vi "AuMT8852B EDER Signal Generator Configuration.vi"(5 "Settings":T1={"Modulation Scheme"=enum."PI4", "Pattern"=enum."PRBS9", "TX/RX frequency"=0.0, "Frequency units"=enum."MHz", "Power (dBm)"=0.0, "RF state"=enum."RF on"} {"Power (dBm)" format="%.2f"}, 7 "Set/Get (Set)":enum16{"Set", "Get"}(ring), 8 "error in (no error)":errorcluster, 11 "VISA session":refnum<visa-resource-name>) -> (0 "error out":errorcluster, 2 "error code":i32, 3 "VISA session out":refnum<visa-resource-name>, 4 "Settings out":T1={"Modulation Scheme"=enum."PI4", "Pattern"=enum."PRBS9", "TX/RX frequency"=0.0, "Frequency units"=enum."MHz", "Power (dBm)"=0.0, "RF state"=enum."RF on"} {"Power (dBm)" format="%.2f"})   [LabVIEW 2017]
doc: "Anritsu MT8852B Bluetooth Tester\n\nConfigures the EDR Signal Generator mode. To enter Signal Generator mode, use the Operation Mode command.\n\nINPUTS\nSet/Get - whether to send or retrieve the parameters.\nSettings - new parameters of the signal generator mode.\n\nINPUTS\nSettings out - current parameters of the signal generator mode."
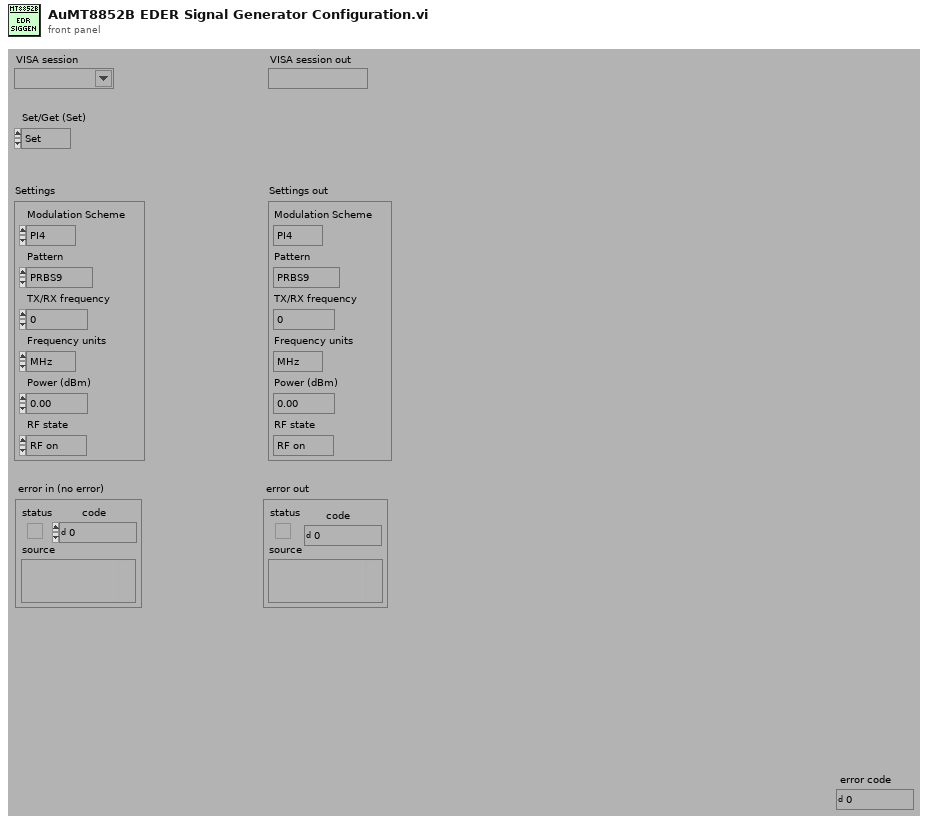
[diagram p1: front panel]
types:
  T1 = cluster{"Modulation Scheme":enum16{"PI4", "8DPSK"}, "Pattern":enum16{"PRBS9", "PRBS15"}, "TX/RX frequency":dbl, "Frequency units":enum16{"Channel", "MHz"}, "Power (dBm)":dbl, "RF state":enum16{"RF off", "RF on"}}
  T2 = enum16{"Simulate", "Range check", "Cache", "Query instrument status"}
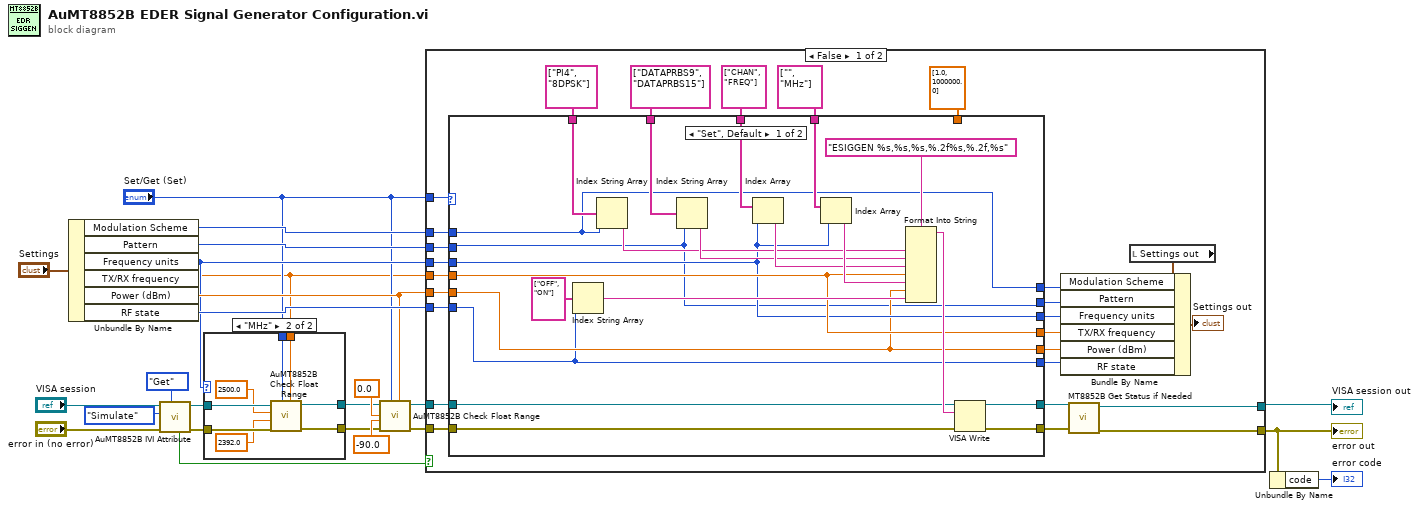
[diagram p0: block diagram]
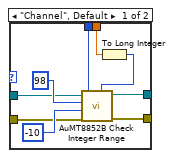
[diagram p2: hidden frame]
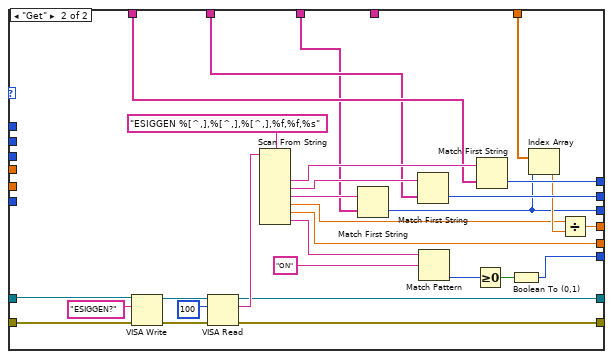
[diagram p3: hidden frame]
diagram:
  n1 = Unbundle By Name("Settings") -> ("Modulation Scheme"=w14:enum16{"PI4", "8DPSK"}, "Pattern"=w13:enum16{"PRBS9", "PRBS15"}, "Frequency units"=w3:enum16{"Channel", "MHz"}, "TX/RX frequency"=w1:dbl, "Power (dBm)"=w11:dbl, "RF state"=w12:enum16{"RF off", "RF on"})
  n2 = call <instrlib>:"AuMT8852B IVI Attribute.vi"("Set/Get (Set)"=enum16{"Set", "Get"}."Get", "error in (no error)"="error in (no error)", "Flag (Simulate)"=T2."Simulate", "VISA session"="VISA session") -> ("error out"=w7:errorcluster, "VISA session out"=w4:refnum<visa-resource-name>, "Value out"=w18:bool)  [unwired: 5 in]
  n3 = case shown="\"MHz\"" w3 {
    tunnel: w7 -> [w31 w41]
    tunnel: [w30 w40] -> w6
    tunnel: [w29 w39] -> w5
    tunnel: w4 -> [w28 w38]
    tunnel: "Set/Get (Set)" -> [w27 w35]
    tunnel: w1 -> [w26 w34]
    frame "Channel", Default {
      n4 = To Long Integer(number=w26) -> (32bit integer=w25:i32)
      n5 = call <instrlib>:"AuMT8852B Check Integer Range.vi"("Value (0)"=w25, "Set/Get (Set)"=w27, "error in (no error)"=w31, "Lower limit (-1)"=-10, "Upper limit (1)"=98, "VISA session"=w28) -> ("error out"=w30:errorcluster, "VISA session out"=w29:refnum<visa-resource-name>)  [unwired: 4 in]
    }
    frame "MHz" {
      n6 = call <instrlib>:"AuMT8852B Check Float Range.vi"("Value (0)"=w34, "Set/Get (Set)"=w35, "error in (no error)"=w41, "Lower limit (-1)"=2392.0, "Upper limit (1)"=2500.0, "VISA session"=w38) -> ("error out"=w40:errorcluster, "VISA session out"=w39:refnum<visa-resource-name>)  [unwired: 4 in]
    }
  }
  n7 = call <instrlib>:"AuMT8852B Check Float Range.vi"("Value (0)"=w11, "Set/Get (Set)"="Set/Get (Set)", "error in (no error)"=w6, "Lower limit (-1)"=-90.0, "Upper limit (1)"=0.0, "VISA session"=w5) -> ("error out"=w17:errorcluster, "VISA session out"=w16:refnum<visa-resource-name>)  [unwired: 4 in]
  n8 = case shown="False" w18 {
    tunnel: [w66 w120] -> w8
    tunnel: [w67 w119] -> w9
    tunnel: w17 -> [w51 w119]
    tunnel: w16 -> [w50 w120]
    tunnel: w3 -> [w49 _]
    tunnel: "Set/Get (Set)" -> [w48 _]
    tunnel: w14 -> [w47 _]
    tunnel: w13 -> [w46 _]
    tunnel: w1 -> [w45 _]
    tunnel: w11 -> [w44 _]
    tunnel: w12 -> [w43 _]
    frame False {
      n9 = case shown="\"Set\", Default" w48 {
        tunnel: [w89 w106] -> w52
        tunnel: [w88 w105] -> w53
        tunnel: [w72 w113] -> w61
        tunnel: [w71 w93] -> w60
        tunnel: [w70 w108] -> w64
        tunnel: [w69 w104] -> w65
        tunnel: string[] ["PI4", "8DPSK"] -> [w76 w96]
        tunnel: string[] ["DATAPRBS9", "DATAPRBS15"] -> [w75 w95]
        tunnel: string[] ["CHAN", "FREQ"] ("Array Constant") -> [w80 w94]
        tunnel: string[] ["", "MHz"] ("Array Constant") -> [w82 _]
        tunnel: [w74 w101] -> w62
        tunnel: dbl[] [1.0, 1000000.0] ("Array Constant") -> [_ w100]
        tunnel: [w73 w90] -> w63
        tunnel: w51 -> [w85 w92]
        tunnel: w50 -> [w84 w91]
        tunnel: w49 -> [w73 _]
        tunnel: w47 -> [w69 _]
        tunnel: w46 -> [w70 _]
        tunnel: w45 -> [w74 _]
        tunnel: w44 -> [w72 _]
        tunnel: w43 -> [w71 _]
        frame "Set", Default {
          n10 = Index String Array(1:w71, 2:string[] ["OFF", "ON"]) -> (0:w83:string)  [unwired: 1 in]
          n11 = Index String Array(1:w69, 2:w76) -> (0:w77:string)  [unwired: 1 in]
          n12 = Index String Array(1:w70, 2:w75) -> (0:w78:string)  [unwired: 1 in]
          n13 = Index Array(array=w80, index=w73) -> (element=w79:string)
          n14 = Index Array(array=w82, index=w73) -> (element=w81:string)
          n15 = Format Into String(format string="ESIGGEN %s,%s,%s,%.2f%s,%.2f,%s" ("Format String"), w77, w78, w79, w74, w81, w72, w83) -> (resulting string=w86:string)  [unwired: 2 in, 1 out]
          n16 = VISA Write(VISA resource name=w84, write buffer=w86, error in (no error)=w85) -> (VISA resource name out=w89:refnum<visa-resource-name>, error out=w88:errorcluster)  [unwired: 1 out]
        }
        frame "Get" {
          n17 = VISA Write(VISA resource name=w91, write buffer="ESIGGEN?" ("write buffer (\"\")"), error in (no error)=w92) -> (VISA resource name out=w115:refnum<visa-resource-name>, error out=w116:errorcluster)  [unwired: 1 out]
          n18 = VISA Read(VISA resource name=w115, byte count=u32 100 ("byte count (0)"), error in (no error)=w116) -> (VISA resource name out=w106:refnum<visa-resource-name>, read buffer=w107:string, error out=w105:errorcluster)  [unwired: 1 out]
          n19 = Scan From String(format string="ESIGGEN %[^,],%[^,],%[^,],%f,%f,%s" ("Format String"), input string=w107) -> (output 1=w99:string, output 2=w98:string, output 3=w97:string, output 4=w102:dbl, output 5=w113:dbl, output 6=w111:string)  [unwired: 8 in, 3 out]
          n20 = Match First String(2:w94, 3:w97) -> (0:w90:i32)  [unwired: 1 out]
          n21 = Match First String(2:w95, 3:w98) -> (0:w108:i32)  [unwired: 1 out]
          n22 = Match Pattern(string=w111, regular expression="ON") -> (offset past match=w110:i32)  [unwired: 1 in, 3 out]
          n23 = Greater Or Equal To 0?(x=w110) -> (x >= 0?=w109:bool)
          n24 = Match First String(2:w96, 3:w99) -> (0:w104:i32)  [unwired: 1 out]
          n25 = Boolean To (0,1)(Boolean=w109) -> (0, 1=w93:i16)
          n26 = Index Array(array=w100, index=w90) -> (element=w103:dbl)
          n27 = Divide(x=w102, y=w103) -> (x/y=w101:dbl)
        }
      }
      n28 = call <instrlib>:"MT8852B Get Status if Needed.vi"("error in (no error)"=w53, "VISA session"=w52) -> ("error out"=w67:errorcluster, "VISA session out"=w66:refnum<visa-resource-name>)  [unwired: 8 in]
      n29 = local read "Settings out"() -> (w56:T1)
      n30 = Bundle By Name(cluster=w56, "Modulation Scheme"=w65, "Pattern"=w64, "Frequency units"=w63, "TX/RX frequency"=w62, "Power (dBm)"=w61, "RF state"=w60) -> (→"Settings out":T1)
    }
    frame True {
    }
  }
  "error out" <- w9
  "VISA session out" <- w8
  n31 = Unbundle By Name(w9) -> ("code"=→"error code":i32)
